vi "motorTorque.vi"(7 "omega":dbl, 9 "Motor":T1={"Ke (V)"=0.0183, "R (ohms)"=0.09, "KT (Nm/A)"=0.0183, "Tf (Nm)"=0.4} {"Tf (Nm)" format="%#_13g"; "KT (Nm/A)" format="%#_13g"; "R (ohms)" format="%#_13g"; "Ke (V)" format="%#_13g"}, 10 "Duty Cycle":dbl) -> (3 "Total Torque":dbl)   [LabVIEW 2016]
panel:
  out "Output Torque":dbl
  out "Current":dbl
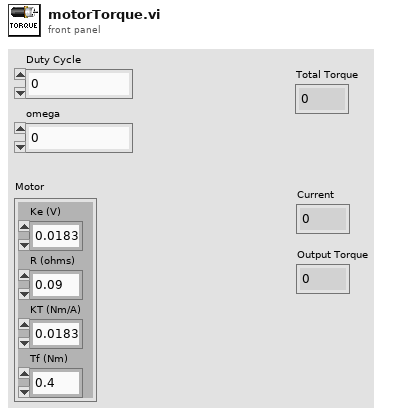
[diagram p1: front panel]
types:
  T1 = cluster{"Ke (V)":dbl, "R (ohms)":dbl, "KT (Nm/A)":dbl, "Tf (Nm)":dbl}
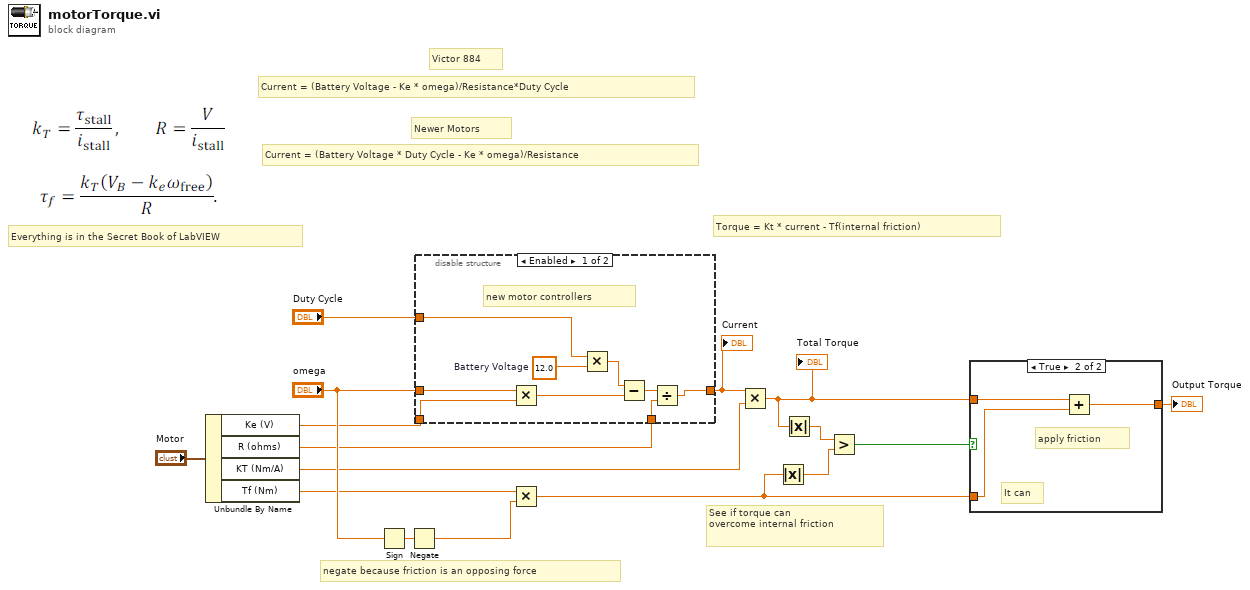
[diagram p0: block diagram]
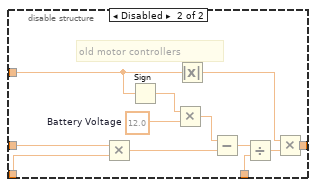
[diagram p2: hidden frame]
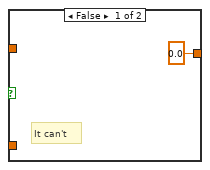
[diagram p3: hidden frame]
diagram:
  # "See if torque can\novercome internal friction"
  # "negate because friction is an opposing force"
  # "Everything is in the Secret Book of LabVIEW"
  # "Torque = Kt * current - Tf(internal friction)"
  # "Current = (Battery Voltage * Duty Cycle - Ke * omega)/Resistance"
  # "Newer Motors"
  # "Current = (Battery Voltage - Ke * omega)/Resistance*Duty Cycle"
  # "Victor 884"
  n1 = Unbundle By Name("Motor") -> ("Ke (V)"=w4:dbl, "R (ohms)"=w3:dbl, "KT (Nm/A)"=w2:dbl, "Tf (Nm)"=w1:dbl)
  n2 = Sign(1:"omega") -> (0:w13:dbl)
  n3 = Negate(x=w13) -> (-x=w12:dbl)
  n4 = disable-structure shown="Enabled" {
    disable-tunnel: "Duty Cycle" -> [w18 w37]
    disable-tunnel: [w17 w29] -> w15
    disable-tunnel: "omega" -> [w21 w28]
    disable-tunnel: w4 -> [w20 w27]
    disable-tunnel: w3 -> [w19 w26]
    frame Enabled {
      w25 = 12.0  # Battery Voltage
      # "new motor controllers"
      n5 = Multiply(x=w21, y=w20) -> (x*y=w23:dbl)
      n6 = Multiply(x=w18, y=w25) -> (x*y=w24:dbl)
      n7 = Subtract(x=w24, y=w23) -> (x-y=w22:dbl)
      n8 = Divide(x=w22, y=w19) -> (x/y=w17:dbl)
    }
    frame Disabled {
      w36 = 12.0  # Battery Voltage
      # "old motor controllers"
      n9 = Multiply(x=w28, y=w27) -> (x*y=w33:dbl)
      n10 = Sign(1:w37) -> (0:w35:dbl)
      n11 = Multiply(x=w35, y=w36) -> (x*y=w34:dbl)
      n12 = Absolute Value(x=w37) -> (abs(x)=w30:dbl)
      n13 = Subtract(x=w34, y=w33) -> (x-y=w32:dbl)
      n14 = Divide(x=w32, y=w26) -> (x/y=w31:dbl)
      n15 = Multiply(x=w30, y=w31) -> (x*y=w29:dbl)
    }
  }
  "Current" <- w15
  n16 = Multiply(x=w1, y=w12) -> (x*y=w11:dbl)
  n17 = Multiply(x=w15, y=w2) -> (x*y=w7:dbl)
  "Total Torque" <- w7
  n18 = Absolute Value(x=w11) -> (abs(x)=w10:dbl)
  n19 = Absolute Value(x=w7) -> (abs(x)=w9:dbl)
  n20 = Greater?(x=w9, y=w10) -> (0:w8:bool)
  n21 = case shown="True" w8 {
    tunnel: w11 -> [_ w41]
    tunnel: w7 -> [_ w40]
    tunnel: [0.0 w39] -> w6
    frame False {
      # "It can't"
    }
    frame True {
      # "It can"
      # "apply friction"
      n22 = Add(x=w40, y=w41) -> (x+y=w39:dbl)
    }
  }
  "Output Torque" <- w6
